vi "backup sandbox.vi"() -> ()   [LabVIEW 2019]
panel:
  out "resulting string":string
  out "string array":string[](array[string])
  in  "delimited string":string
  out "array w/ subset deleted":string[](array[string])
  out "deleted portion":string[](array[string])
  in  "length":i32
  in  "Array":string[](array[string])
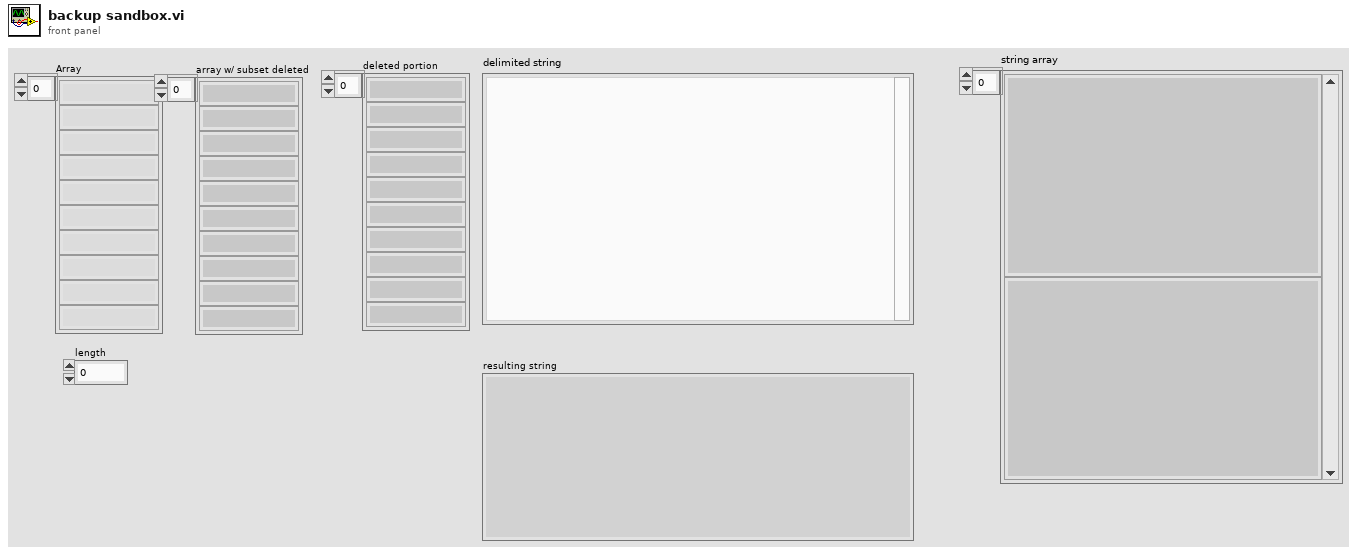
[diagram p1: front panel]
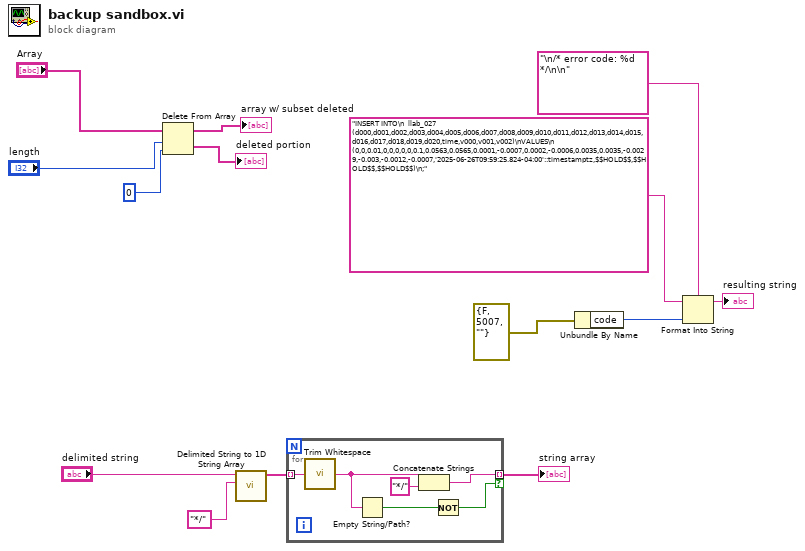
[diagram p0: block diagram]
diagram:
  n1 = Delete From Array(array="Array", length="length", index=0) -> (deleted portion=→"deleted portion":string[], array with subset deleted=→"array w/ subset deleted":string[])
  n2 = call <vilib>:"Delimited String to 1D String Array.vi"("delimiter"="*/", "delimited string"="delimited string") -> ("string array"=w7:string[])  [unwired: 9 in]
  n3 = for {
    tunnel: w7 -> [w19] mode=indexing
    tunnel: [w20] -> w6 mode=indexing if=w15
    n4 = call <vilib>:"Trim Whitespace.vi"("string"=w19) -> ("trimmed string"=w18:string)  [unwired: 1 in]
    n5 = Empty String/Path?(string/path=w18) -> (empty?=w16:bool)
    n6 = Concatenate Strings(w18, "*/" ("string")) -> (w20:string)
    n7 = Not(x=w16) -> (.not. x?=w15:bool)
  }
  "string array" <- w6
  n8 = Unbundle By Name(errorcluster {"status"=FALSE, "code"=5007, "source"=""} ("input cluster")) -> ("code"=w5:i32)
  n9 = Format Into String(format string="\n/* error code: %d */\n\n", initial string="INSERT INTO\n  llab_027 (d000,d001,d002,d003,d004,d005,d006,d007,d008,d009,d010,d011,d012,d013,d014,d015,d016,d017,d018,d019,d020,time,v000,v001,v002)\nVALUES\n  (0,0,0.01,0,0,0,0,0,0.1,0.0563,0.0565,0.0001,-0.0007,0.0002,-0.0006,0.0035,0.0035,-0.0029,-0.003,-0.0012,-0.0007,'2025-06-26T09:59:25.824-04:00'::timestamptz,$$HOLD$$,$$HOLD$$,$$HOLD$$)\n;", w5) -> (resulting string=→"resulting string":string)  [unwired: 1 in, 1 out]
